vi "conv2matV2.vi"(0 "Ref Num":refnum<file>, 1 "Array name":string, 7 "pos offset (bytes:0)":i32, 11 "error in (no error)":errorcluster, 12 "1D-array":dbl[](array[numeric]) min=0.0 max=127.0 format="%.2f") -> (4 "Dup Ref Num":refnum<file>, 8 "mark after write (bytes)":i32, 15 "error out":errorcluster)   [LabVIEW 2015]
doc: "CONV2MAT.VI exports an array to Matlab format (.MAT file) at the specified location. The default location is at the end of file. The user will have to open the output file before and close it afterwards. The VI does incoming and internal error checking and does not write if an incoming error occurs.\n\nConnect the following terminals:\n- Ref number\n- array name; this name will also apear when the resulting file is read\n into Matlab.\n- Data type; this specifies the output data type. This can come in\n handy if you want to reduce the output file size.\n- either 1D-array, 2D-array or String. If you want to write a string,\n do not connect Data Type (caracters will be converted to floating\n point numbers representing their ASCII-value).\n\nPos mode and Pos offset default to write any data at the end of the file.\n\nAlbert K. Wijnja\nUniversity of Technology Eindhoven\nE-mail: albert@wfw.wtb.tue.nl\n\nSeptember 1994"
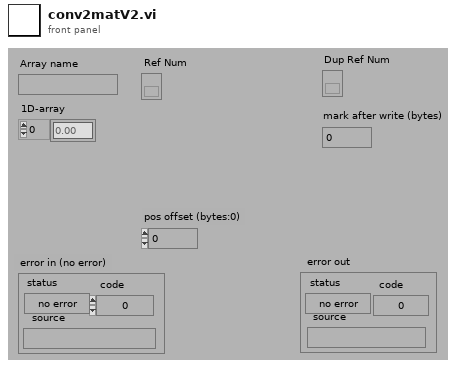
[diagram p1: front panel]
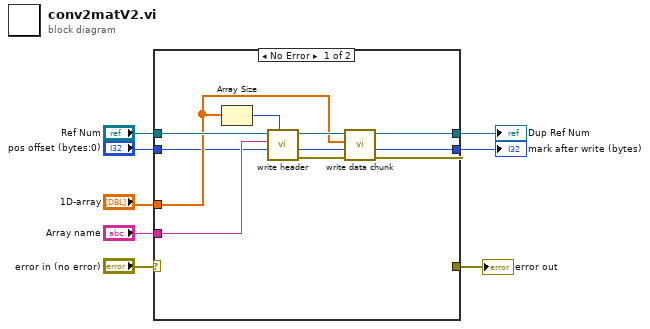
[diagram p0: block diagram]
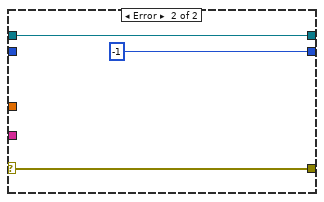
[diagram p2: hidden frame]
diagram:
  n1 = case shown="No Error" "error in (no error)" {
    selector: "error in (no error)" -> [_ w20]
    tunnel: [w10 w20] -> w8
    tunnel: [w17 w22] -> w6
    tunnel: "Ref Num" -> [w19 w22]
    tunnel: [w11 -1] -> w5
    tunnel: "1D-array" -> [w14 _]
    tunnel: "Array name" -> [w16 _]
    tunnel: "pos offset (bytes:0)" -> [w9 _]
    frame No Error {
      n2 = Array Size(array=w14) -> (size(s)=w15:i32)
      n3 = call "write header.vi"("number of samples for this channel"=w15, "pos offset (bytes:0)"=w9, "Channel name"=w16, "Ref Num"=w19) -> ("error out"=w13:errorcluster, "mark after write (bytes)"=w12:i32, "Dup Ref Num"=w18:refnum<file>)  [unwired: 5 in]
      n4 = call "write data chunk.vi"("error in (no error)"=w13, "pos offset (bytes:0)"=w12, "1D-array (chunk)"=w14, "Ref Num"=w18) -> ("error out"=w10:errorcluster, "mark after write (bytes)"=w11:i32, "Dup Ref Num"=w17:refnum<file>)  [unwired: 5 in]
    }
    frame Error {
    }
  }
  "Dup Ref Num" <- w6
  "error out" <- w8
  "mark after write (bytes)" <- w5
